vi "fifo2file.vi"(11 "DataLoggingParam":T1={"Fifo Size"=0, "FileRefnum"=refnum, "FifoRefnum"=refnum, "Fifo Time Out (ms)"=500, "MaxNumFileWrite"=255, "Force Num Array"=0}) -> (1 "fifo full counter":u16, 3 "DataLoggingParam 2":T1={"Fifo Size"=0, "FileRefnum"=refnum, "FifoRefnum"=refnum, "Fifo Time Out (ms)"=500, "MaxNumFileWrite"=255, "Force Num Array"=0})   [LabVIEW 2010, in "kevLib2011.lvlib"]
uses:
  kevLib2011.lvlib
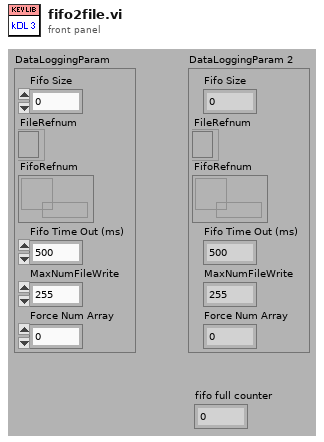
[diagram p1: front panel]
types:
  T1 = cluster{"Fifo Size":u32, "FileRefnum":refnum<file>, "FifoRefnum":refnum<k33>, "Fifo Time Out (ms)":i32, "MaxNumFileWrite":i32, "Force Num Array":i32}
  T2 = enum16{"big-endian, network order", "native, host order", "little-endian"}
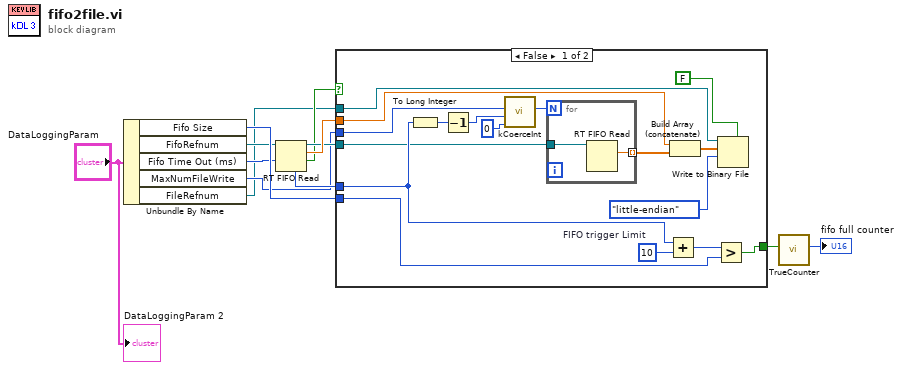
[diagram p0: block diagram]
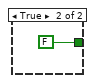
[diagram p2: hidden frame]
diagram:
  n1 = Unbundle By Name("DataLoggingParam") -> ("Fifo Size"=w5:u32, "FifoRefnum"=w4:refnum<k33>, "Fifo Time Out (ms)"=w3:i32, "MaxNumFileWrite"=w2:i32, "FileRefnum"=w1:refnum<file>)
  n2 = RT FIFO Read(0:w4, 2:w3) -> (7:w12:u32, 8:w10:refnum<k33>, 9:w11:dbl, 10:w9:bool)  [unwired: 2 in, 1 out]
  n3 = case shown="False" w9 {
    tunnel: [w29 FALSE] -> w7
    tunnel: w12 -> [w26 _]
    tunnel: w11 -> [w23 _]
    tunnel: w10 -> [w22 _]
    tunnel: w5 -> [w15 _]
    tunnel: w2 -> [w14 _]
    tunnel: w1 -> [w13 _]
    frame False {
      w27 = u32 10  # FIFO trigger Limit
      n4 = To Long Integer(number=w26) -> (32bit integer=w19:i32)
      n5 = Decrement(x=w19) -> (x-1=w18:i32)
      n6 = call "kCoerceInt.vi"("lower"=0 ("lower limit"), "input"=w18, "upper"=w14) -> ("output"=w16:i32)  [unwired: 7 in, 1 out]
      n7 = for {
        N: w16 -> [_]
        tunnel: w22 -> [w31]
        tunnel: [w30] -> w24 mode=indexing
        n8 = RT FIFO Read(0:w31) -> (9:w30:dbl)  [unwired: 2 in, 5 out]
      }
      n9 = Add(x=w26, y=w27) -> (x+y=w28:u32)
      n10 = Build Array (concatenate)(w23, w24) -> (w25:dbl[])
      n11 = Greater?(x=w28, y=w15) -> (0:w29:bool)
      n12 = Write to Binary File(file (use dialog)=w13, data=w25, 5:FALSE ("prepend array or string size? (T)"), 9:T2."little-endian" ("byte order (0:big-endian, network order)")) -> ()  [unwired: 1 in, 4 out]
    }
    frame True {
    }
  }
  n13 = call "TrueCounter.vi"("True?"=w7) -> ("True Count"=→"fifo full counter":u16)  [unwired: 9 in]
  "DataLoggingParam 2" <- "DataLoggingParam"
